vi "Create Channel Labels.vi"(8 "error in":errorcluster, 11 "DIG_IO in":refnum<class "DIG_IO.lvclass">) -> (0 "error out":errorcluster, 3 "DIG_IO out":refnum<class "DIG_IO.lvclass">)   [LabVIEW 2019, in "DIG_IO.lvlib" / "DIG_IO.lvclass"]
uses:
  Library/DIG_IO.lvclass
  Library/DIG_IO.lvclass/DIG_IO.ctl
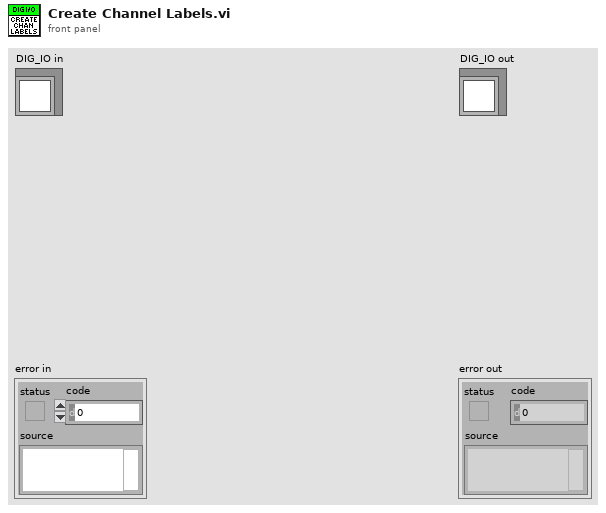
[diagram p1: front panel]
types:
  T1 = enum8{"Enabled", "Disabled", "Disabled and Grayed Out"}
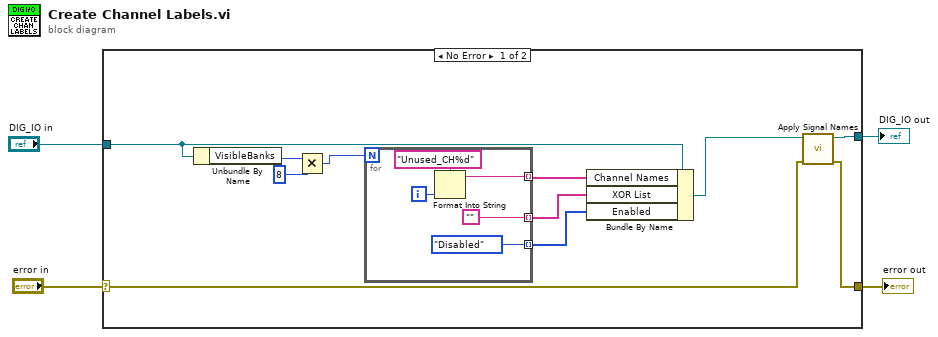
[diagram p0: block diagram]
diagram:
  n1 = case shown="No Error" "error in" {
    selector: "error in" -> [w14 w22]
    tunnel: [w13 w22] -> w3
    tunnel: [w15 w21] -> w1
    tunnel: "DIG_IO in" -> [w11 w21]
    frame No Error {
      n2 = Unbundle By Name(w11) -> ("VisibleBanks"=w7:u8)
      n3 = Multiply(x=w7, y=u8 8) -> (x*y=w5:u8)
      n4 = for {
        N: w5 -> [_]
        tunnel: [w18] -> w10 mode=indexing
        tunnel: [""] -> w9 mode=indexing
        tunnel: [T1."Disabled" ("element")] -> w8 mode=indexing
        i -> [w20]
        n5 = Format Into String(format string="Unused_CH%d", w20) -> (resulting string=w18:string)  [unwired: 2 in, 1 out]
      }
      n6 = Bundle By Name(cluster=w11, "Channel Names"=w10, "XOR List"=w9, "Enabled"=w8) -> (w12:refnum<class "DIG_IO.lvclass">)
      n7 = call "Apply Signal Names.vi"("error in"=w14, "DIG_IO in"=w12) -> ("error out"=w13:errorcluster, "DIG_IO out"=w15:refnum<class "DIG_IO.lvclass">)  [unwired: 8 in]
    }
    frame Error {
    }
  }
  "error out" <- w3
  "DIG_IO out" <- w1
